vi "Find Safe Path.vi"(6 "Include Start":bool=TRUE, 7 "error in":errorcluster, 9 "Destination":string, 10 "Gantry in":refnum<class "Gantry.lvclass">) -> (0 "error out":errorcluster, 1 "Point Names":string[](array[string]), 2 "Points Array":refnum<class "Vec3d.lvclass">[](array[class]), 3 "Gantry out":refnum<class "Gantry.lvclass">)   [LabVIEW 2023, in "Gantry.lvclass"]
uses:
  Gantry.lvclass
  Vec3d Class/Vec3d.lvclass
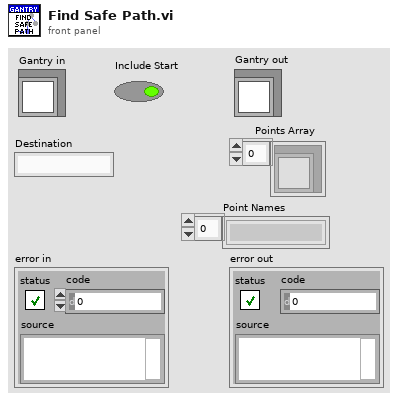
[diagram p1: front panel]
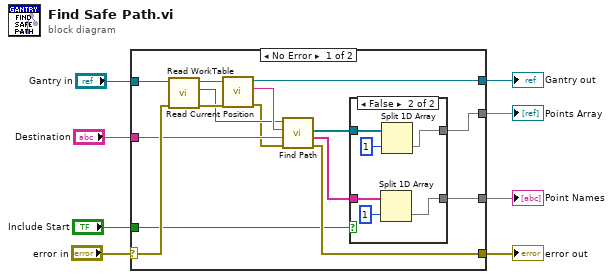
[diagram p0: block diagram]
diagram:
  n1 = case shown="No Error" "error in" {
    selector: "error in" -> [w20 w33]
    tunnel: [w23 w32] -> w8
    tunnel: "Destination" -> [w17 _]
    tunnel: "Gantry in" -> [w22 w32]
    tunnel: [w14 w33] -> w4
    tunnel: [w12 _] -> w3
    tunnel: "Include Start" -> [w11 _]
    tunnel: [w9 _] -> w1
    frame No Error {
      n2 = call-dynamic "Read WorkTable.vi"("error in"=w20, "Gantry Class in"=w22) -> ("error out"=w21:errorcluster, "Worktable"=w16:refnum<class "FlexWorktable.lvclass">, "Gantry Class out"=w19:refnum<class "Gantry.lvclass">)  [unwired: 7 in]
      n3 = call-dynamic "Read Current Position.vi"("error in"=w21, "Gantry in"=w19) -> ("error out"=w15:errorcluster, "Current Position"=w18:string, "Gantry out"=w23:refnum<class "Gantry.lvclass">)  [unwired: 7 in]
      n4 = call "Find Path.vi"("error in"=w15, "end"=w17, "start"=w18, "FlexWorktable in"=w16) -> ("error out"=w14:errorcluster, "Point Names"=w10:string[], "Points"=w13:refnum<class "Vec3d.lvclass">[])  [unwired: 4 in, 1 out]
      n5 = case shown="False" w11 {
        tunnel: w13 -> [w25 w31]
        tunnel: [w25 w29] -> w12
        tunnel: w10 -> [w24 w27]
        tunnel: [w24 w26] -> w9
        frame True {
        }
        frame False {
          n6 = Split 1D Array(array=w27, index=1) -> (second subarray=w26:string[])  [unwired: 1 out]
          n7 = Split 1D Array(array=w31, index=1) -> (second subarray=w29:refnum<class "Vec3d.lvclass">[])  [unwired: 1 out]
        }
      }
    }
    frame Error {
    }
  }
  "error out" <- w4
  "Points Array" <- w3
  "Gantry out" <- w8
  "Point Names" <- w1
